vi "ExecuteMove.vi"(6 "Long Castle?":bool, 8 "Small Castle?":bool, 9 "In the Passage?":bool, 10 "Last Square?":bool, 11 "Input DataBase":T5) -> (3 "Output Squares":T1[][](array[typedef]))   [LabVIEW 2019]
uses:
  #typedef_DataBase.ctl
  #typedef_SquareType.ctl
  #typedef_Color.ctl
  #typedef_Piece.ctl
  #typedef_PieceType.ctl
  #typedef_SquareLook.ctl
  #typedef_SpecialMoves.ctl
panel:
  out "?":u16[][](array[ring])
  out "?":u16[][](array[ring])
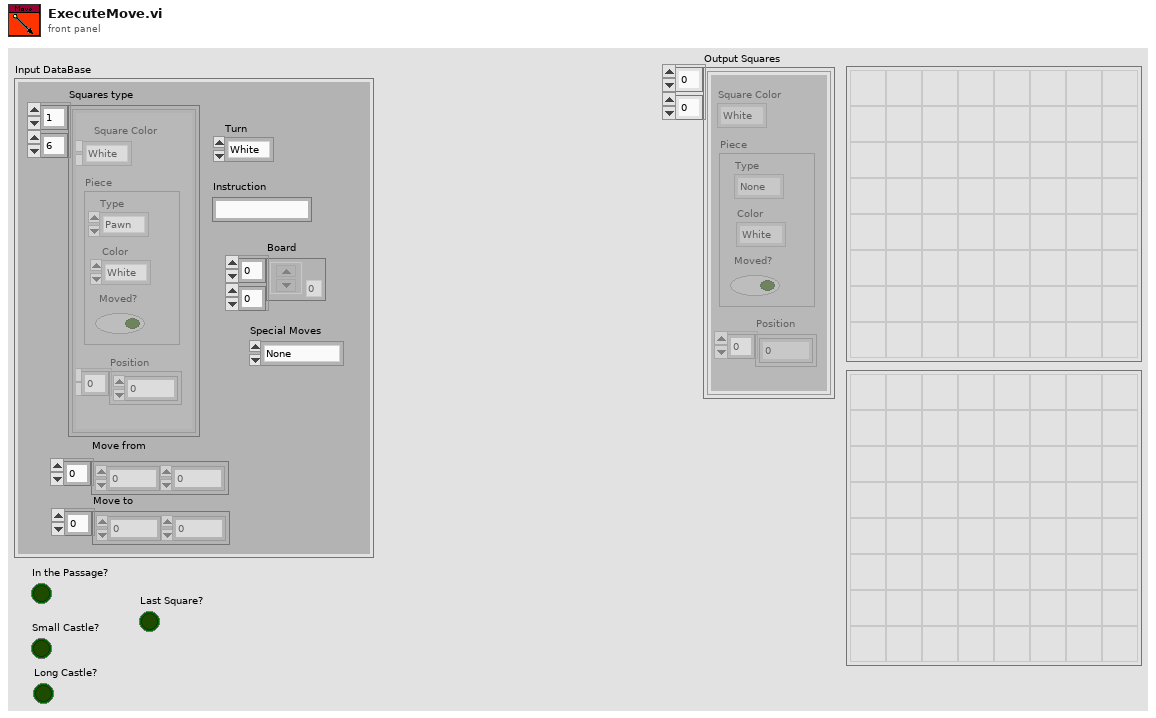
[diagram p1: front panel]
types:
  T1 = typedef "#typedef_SquareType.ctl" = cluster{"Square Color":T2, "Position":i32[], "Piece":T3}
  T2 = typedef "#typedef_Color.ctl" = enum16{"White", "Black"}
  T3 = typedef "#typedef_Piece.ctl" = cluster{"Type":T4, "Color":T2, "Moved?":bool}
  T4 = typedef "#typedef_PieceType.ctl" = enum16{"None", "Pawn", "Knight", "Bishop", "Rook", "Queen", "King"}
  T5 = typedef "#typedef_DataBase.ctl" = cluster{"Squares type":T1[][], "Turn":T2, "Move from":i32[], "Move to":i32[], "Instruction":string, "Board":T6[][], "Special Moves":T7}
  T6 = typedef "#typedef_SquareLook.ctl" = u16
  T7 = typedef "#typedef_SpecialMoves.ctl" = enum16{"None", "Last Square", "Beat in the Passage", "Short Castle", "Long Castle"}
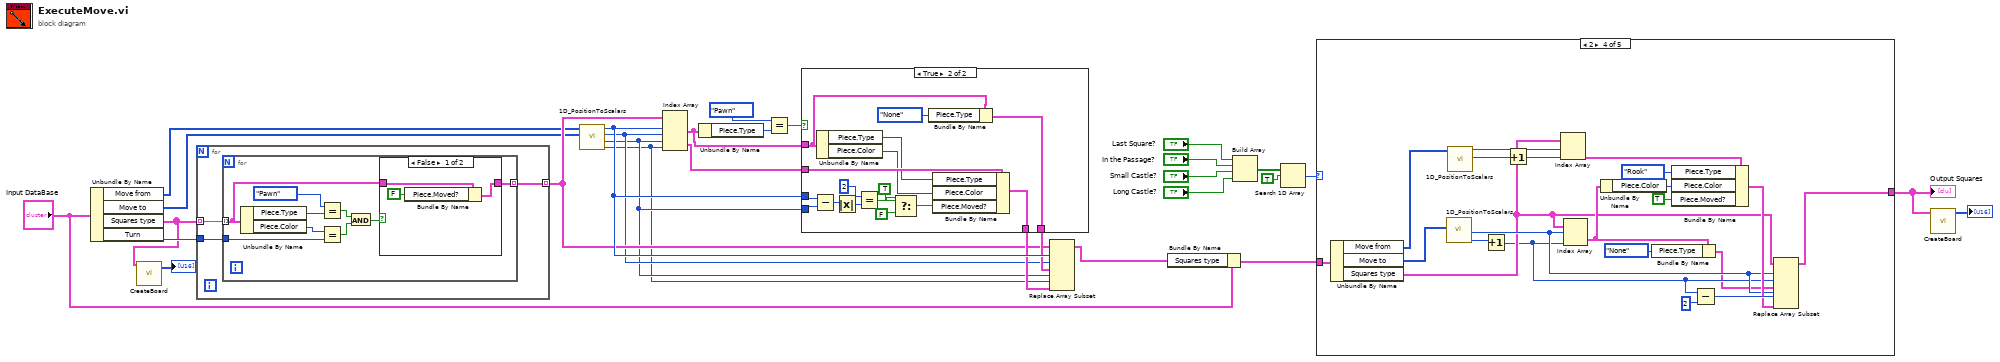
[diagram p0: block diagram]
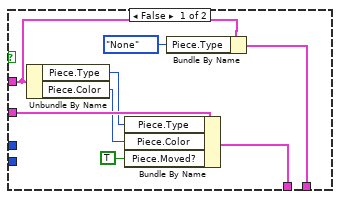
[diagram p3: hidden frame]
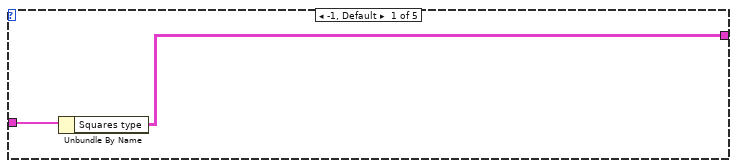
[diagram p4: hidden frame]
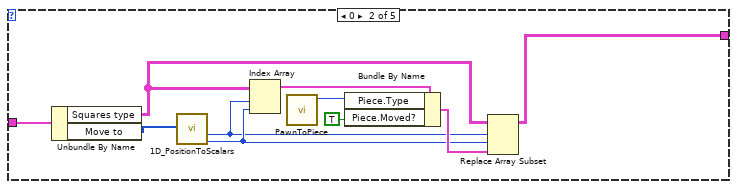
[diagram p5: hidden frame]
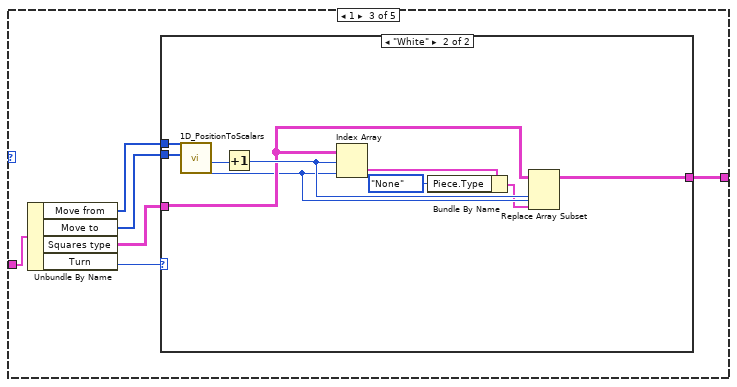
[diagram p6: hidden frame]
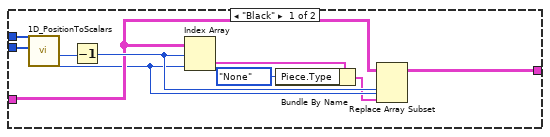
[diagram p7: hidden frame]
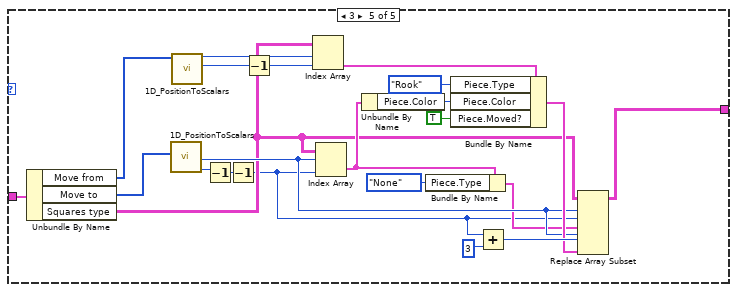
[diagram p8: hidden frame]
diagram:
  n1 = Unbundle By Name("Input DataBase") -> ("Move from"=w17:i32[], "Move to"=w16:i32[], "Squares type"=w6:T1[][], "Turn"=w19:T2)
  n2 = call "CreateBoard.vi"("Squares type"=w6) -> ("Board"=→"?":u16[][])  [unwired: 10 in]
  n3 = for {
    tunnel: w6 -> [w32] mode=indexing
    tunnel: w19 -> [w31]
    tunnel: [w30] -> w18 mode=indexing
    n4 = for {
      tunnel: w32 -> [w34] mode=indexing
      tunnel: w31 -> [w40]
      tunnel: [w33] -> w30 mode=indexing
      n5 = Unbundle By Name(w34) -> ("Piece.Type"=w39:T4, "Piece.Color"=w41:T2)
      n6 = Equal?(x=#typedef_PieceType."Pawn", y=w39) -> (x = y?=w37:bool)
      n7 = Equal?(x=w41, y=w40) -> (x = y?=w36:bool)
      n8 = And(x=w37, y=w36) -> (x .and. y?=w35:bool)
      n9 = case shown="False" w35 {
        tunnel: w34 -> [w44 w45]
        tunnel: [w42 w45] -> w33
        frame False {
          n10 = Bundle By Name(cluster=w44, "Piece.Moved?"=FALSE) -> (w42:T1)
        }
        frame True {
        }
      }
    }
  }
  n11 = call "1D_PositionToScalars.vi"("Move to"=w16, "Move from"=w17) -> ("Column to"=w13:i32, "Row to"=w14:i32, "Column from"=w15:i32, "Row from"=w29:i32)  [unwired: 6 in]
  n12 = Index Array(array=w18, index (row) #1=w29, index (col) #1=w15, index (row) #2=w14, index (col) #2=w13) -> (element #1=w26:T1, element #2=w25:T1)
  n13 = Unbundle By Name(w26) -> ("Piece.Type"=w22:T4)
  n14 = Equal?(x=#typedef_PieceType."Pawn", y=w22) -> (x = y?=w24:bool)
  n15 = case shown="True" w24 {
    tunnel: w25 -> [w53 w69]
    tunnel: w26 -> [w48 w65]
    tunnel: [w47 w64] -> w27
    tunnel: [w46 w63] -> w28
    tunnel: w29 -> [_ w62]
    tunnel: w14 -> [_ w61]
    frame False {
      n16 = Unbundle By Name(w48) -> ("Piece.Type"=w52:T4, "Piece.Color"=w51:T2)
      n17 = Bundle By Name(cluster=w53, "Piece.Type"=w52, "Piece.Color"=w51, "Piece.Moved?"=TRUE) -> (w46:T1)
      n18 = Bundle By Name(cluster=w48, "Piece.Type"=#typedef_PieceType."None") -> (w47:T1)
    }
    frame True {
      n19 = Subtract(x=w62, y=w61) -> (x-y=w60:i32)
      n20 = Unbundle By Name(w65) -> ("Piece.Type"=w68:T4, "Piece.Color"=w67:T2)
      n21 = Absolute Value(x=w60) -> (abs(x)=w59:i32)
      n22 = Equal?(x=2, y=w59) -> (x = y?=w57:bool)
      n23 = Select(t=TRUE, s=w57, f=FALSE) -> (s? t:f=w54:bool)
      n24 = Bundle By Name(cluster=w65, "Piece.Type"=#typedef_PieceType."None") -> (w64:T1)
      n25 = Bundle By Name(cluster=w69, "Piece.Type"=w68, "Piece.Color"=w67, "Piece.Moved?"=w54) -> (w63:T1)
    }
  }
  n26 = Replace Array Subset(array=w18, new element #1=w27, index (row) #1=w29, index (col) #1=w15, new element #2=w28, index (row) #2=w14, index (col) #2=w13) -> (w11:T1[][])
  n27 = Bundle By Name(cluster="Input DataBase", "Squares type"=w11) -> (w10:T5)
  n28 = Build Array("Last Square?", "In the Passage?", "Small Castle?", "Long Castle?") -> (w5:bool[])
  n29 = Search 1D Array(1D array=w5, element=TRUE) -> (index of element=w21:i32)  [unwired: 1 in]
  n30 = case shown="2" w21 {
    tunnel: w10 -> [w71 w81 w83 w119 w141]
    tunnel: [w70 w74 w82 w113 w135] -> w9
    frame -1, Default {
      n31 = Unbundle By Name(w71) -> ("Squares type"=w70:T1[][])
    }
    frame 0 {
      n32 = Unbundle By Name(w81) -> ("Squares type"=w76:T1[][], "Move to"=w80:i32[])
      n33 = call "1D_PositionToScalars.vi"("Move to"=w80) -> ("Column to"=w73:i32, "Row to"=w72:i32)  [unwired: 7 in, 2 out]
      n34 = Index Array(array=w76, index (row)=w72, index (col)=w73) -> (element=w79:T1)
      n35 = call "PawnToPiece.vi"() -> ("Figure type"=w78:T4)  [unwired: 11 in]
      n36 = Bundle By Name(cluster=w79, "Piece.Type"=w78, "Piece.Moved?"=TRUE) -> (w75:T1)
      n37 = Replace Array Subset(array=w76, new element=w75, index (row)=w72, index (col)=w73) -> (w74:T1[][])
    }
    frame 1 {
      n38 = Unbundle By Name(w83) -> ("Move from"=w85:i32[], "Move to"=w84:i32[], "Squares type"=w86:T1[][], "Turn"=w87:T2)
      n39 = case shown="\"White\"" w87 {
        tunnel: w86 -> [w93 w103]
        tunnel: w85 -> [w92 w102]
        tunnel: w84 -> [w91 w101]
        tunnel: [w88 w98] -> w82
        frame "Black" {
          n40 = call "1D_PositionToScalars.vi"("Move to"=w91, "Move from"=w92) -> ("Column to"=w90:i32, "Row to"=w95:i32)  [unwired: 6 in, 2 out]
          n41 = Decrement(x=w95) -> (x-1=w94:i32)
          n42 = Index Array(array=w93, index (row)=w94, index (col)=w90) -> (element=w97:T1)
          n43 = Bundle By Name(cluster=w97, "Piece.Type"=#typedef_PieceType."None") -> (w89:T1)
          n44 = Replace Array Subset(array=w93, new element=w89, index (row)=w94, index (col)=w90) -> (w88:T1[][])
        }
        frame "White" {
          n45 = call "1D_PositionToScalars.vi"("Move to"=w101, "Move from"=w102) -> ("Column to"=w100:i32, "Row to"=w105:i32)  [unwired: 6 in, 2 out]
          n46 = Increment(x=w105) -> (x+1=w104:i32)
          n47 = Index Array(array=w103, index (row)=w104, index (col)=w100) -> (element=w107:T1)
          n48 = Bundle By Name(cluster=w107, "Piece.Type"=#typedef_PieceType."None") -> (w99:T1)
          n49 = Replace Array Subset(array=w103, new element=w99, index (row)=w104, index (col)=w100) -> (w98:T1[][])
        }
      }
    }
    frame 2 {
      n50 = Unbundle By Name(w119) -> ("Move from"=w118:i32[], "Move to"=w117:i32[], "Squares type"=w114:T1[][])
      n51 = call "1D_PositionToScalars.vi"("Move to"=w117) -> ("Column to"=w116:i32, "Row to"=w115:i32)  [unwired: 7 in, 2 out]
      n52 = call "1D_PositionToScalars.vi"("Move from"=w118) -> ("Column from"=w109:i32, "Row from"=w110:i32)  [unwired: 7 in, 2 out]
      n53 = Increment(x=w116) -> (x+1=w112:i32)
      n54 = Increment(x=w109) -> (x+1=w108:i32)
      n55 = Index Array(array=w114, index (row)=w110, index (col)=w108) -> (element=w123:T1)
      n56 = Index Array(array=w114, index (row)=w115, index (col)=w112) -> (element=w127:T1)
      n57 = Unbundle By Name(w127) -> ("Piece.Color"=w126:T2)
      n58 = Bundle By Name(cluster=w127, "Piece.Type"=#typedef_PieceType."None") -> (w111:T1)
      n59 = Bundle By Name(cluster=w123, "Piece.Type"=#typedef_PieceType."Rook", "Piece.Color"=w126, "Piece.Moved?"=TRUE) -> (w120:T1)
      n60 = Subtract(x=w112, y=2) -> (x-y=w121:i32)
      n61 = Replace Array Subset(array=w114, new element #1=w111, index (row) #1=w115, index (col) #1=w112, new element #2=w120, index (row) #2=w115, index (col) #2=w121) -> (w113:T1[][])
    }
    frame 3 {
      n62 = Unbundle By Name(w141) -> ("Move from"=w140:i32[], "Move to"=w139:i32[], "Squares type"=w136:T1[][])
      n63 = call "1D_PositionToScalars.vi"("Move to"=w139) -> ("Column to"=w138:i32, "Row to"=w137:i32)  [unwired: 7 in, 2 out]
      n64 = call "1D_PositionToScalars.vi"("Move from"=w140) -> ("Column from"=w131:i32, "Row from"=w132:i32)  [unwired: 7 in, 2 out]
      n65 = Decrement(x=w138) -> (x-1=w134:i32)
      n66 = Decrement(x=w134) -> (x-1=w129:i32)
      n67 = Decrement(x=w131) -> (x-1=w130:i32)
      n68 = Index Array(array=w136, index (row)=w132, index (col)=w130) -> (element=w145:T1)
      n69 = Index Array(array=w136, index (row)=w137, index (col)=w129) -> (element=w149:T1)
      n70 = Unbundle By Name(w149) -> ("Piece.Color"=w148:T2)
      n71 = Bundle By Name(cluster=w149, "Piece.Type"=#typedef_PieceType."None") -> (w133:T1)
      n72 = Bundle By Name(cluster=w145, "Piece.Type"=#typedef_PieceType."Rook", "Piece.Color"=w148, "Piece.Moved?"=TRUE) -> (w142:T1)
      n73 = Add(x=w129, y=3) -> (x+y=w143:i32)
      n74 = Replace Array Subset(array=w136, new element #1=w133, index (row) #1=w137, index (col) #1=w129, new element #2=w142, index (row) #2=w137, index (col) #2=w143) -> (w135:T1[][])
    }
  }
  "Output Squares" <- w9
  n75 = call "CreateBoard.vi"("Squares type"=w9) -> ("Board"=→"?":u16[][])  [unwired: 10 in]
